vi "Get Malleable VI Library Info.vi"(8 "error in (no error)":errorcluster, 10 "Malleable VI Name":string, 11 "Library Ref":refnum<vi>) -> (0 "error out":errorcluster, 1 "Malleable VI Path":path, 2 "Found?":bool, 3 "Owner":refnum<vi>)   [LabVIEW 2020]
doc: "Searches the referenced library for the malleable VI."
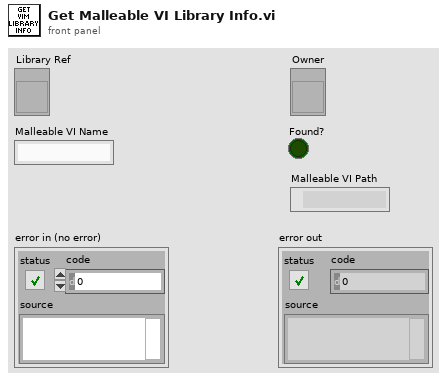
[diagram p1: front panel]
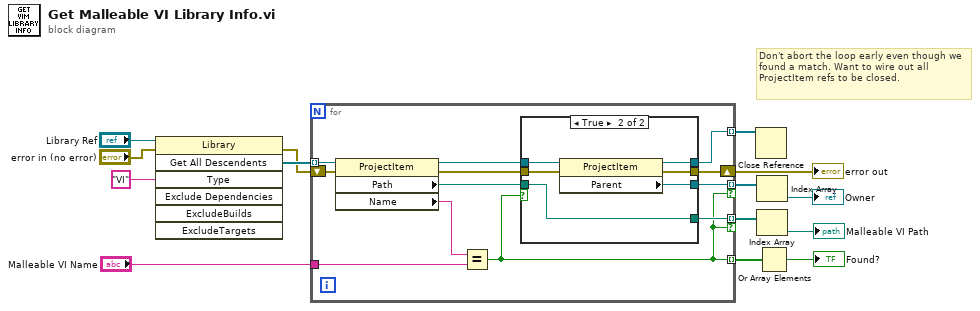
[diagram p0: block diagram]
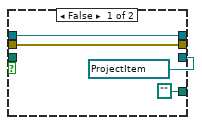
[diagram p2: hidden frame]
diagram:
  # "Don't abort the loop early even though we found a match. Want to wire out all ProjectItem refs to be closed."
  n1 = invoke class="Library" method="Get All Descendents"(reference="Library Ref", error in="error in (no error)", "Type"="VI") -> (error out=w6:errorcluster, "All Descendents"=w13:refnum<vi>[])  [unwired: 4 in, 5 out]
  n2 = for {
    tunnel: w13 -> [w26] mode=indexing
    tunnel: [w23] -> w10 mode=indexing if=w16
    tunnel: "Malleable VI Name" -> [w24]
    tunnel: [w16] -> w9 mode=indexing
    shift-right: [w19] -> w5
    shift-left: w6 -> [w21]
    tunnel: [w17] -> w3 mode=indexing if=w16
    tunnel: [w15] -> w1 mode=indexing
    n3 = property class="ProjectItem"(reference=w26, error in=w21) -> (reference out=w22:refnum<vi>, error out=w20:errorcluster, "Path"=w18:path, "Name"=w25:string)
    n4 = Equal?(x=w25, y=w24) -> (x = y?=w16:bool)
    n5 = case shown="True" w16 {
      tunnel: [refnum<vi> refnum ("Parent") w35] -> w23
      tunnel: w22 -> [w28 w36]
      tunnel: w20 -> [w27 w34]
      tunnel: [w27 w32] -> w19
      tunnel: w18 -> [_ w33]
      tunnel: [path "" w33] -> w17
      tunnel: [w28 w31] -> w15
      frame False {
      }
      frame True {
        n6 = property class="ProjectItem"(reference=w36, error in=w34) -> (reference out=w31:refnum<vi>, error out=w32:errorcluster, "Parent"=w35:refnum<vi>)
      }
    }
  }
  "error out" <- w5
  n7 = Close Reference(reference=w1) -> ()  [unwired: 1 in, 1 out]
  n8 = Index Array(array=w10) -> (element=→"Owner":refnum<vi>)  [unwired: 1 in]
  n9 = Index Array(array=w3) -> (element=→"Malleable VI Path":path)  [unwired: 1 in]
  n10 = Or Array Elements(Boolean array=w9) -> (logical OR=→"Found?":bool)
